vi "Destroy.vi"(8 "error in (no error)":errorcluster, 11 "reference in":refnum<class "GetCostVisitor.lvclass">) -> (0 "error out":errorcluster, 3 "reference out":refnum<class "GetCostVisitor.lvclass">)   [LabVIEW 2020, in "GetCostVisitor.lvclass"]
uses:
  GetCostVisitor.lvclass
  EquipmentVisitor_class/EquipmentVisitor.lvclass
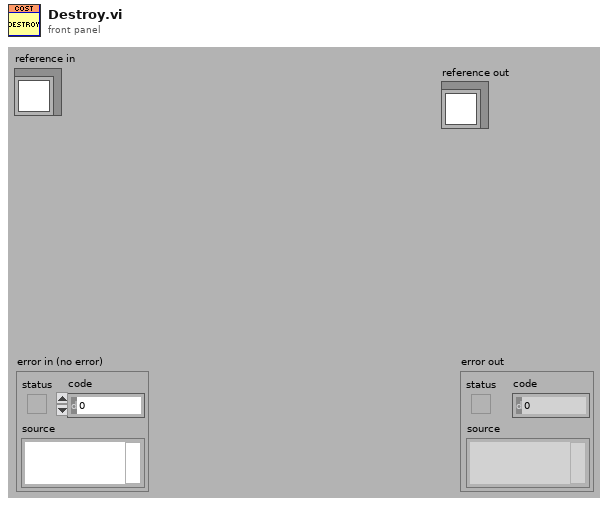
[diagram p1: front panel]
types:
  T1 = typedef "GetCostVisitor.lvclass/ObjectAttributes.ctl" = cluster{"None":bool}
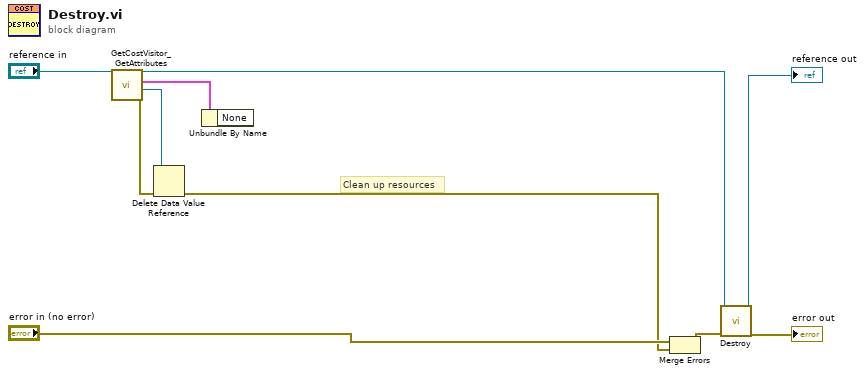
[diagram p0: block diagram]
diagram:
  # "Clean up resources"
  n1 = call "GetCostVisitor_GetAttributes.vi"("reference in"="reference in") -> ("error out"=w7:errorcluster, "DataRef"=w3:refnum<data-value>, "Data"=w6:T1, "reference out"=w4:refnum<class "GetCostVisitor.lvclass">)  [unwired: 7 in]
  n2 = Delete Data Value Reference(data value reference=w3, error in=w7) -> (error out=w1:errorcluster)  [unwired: 1 out]
  n3 = Unbundle By Name(w6) -> ()  [unwired: 1 out]
  n4 = Merge Errors("error in (no error)", w1) -> (w10:errorcluster)
  n5 = call-parent "Destroy.vi"("error in (no error)"=w10, "reference in"=w4) -> ("error out"=→"error out":errorcluster, "reference out"=→"reference out":refnum<class "GetCostVisitor.lvclass">)  [unwired: 8 in]
